vi "VIAn_EasyAnalyze.vi"(8 "error in (no error)":errorcluster, 11 "CommandLine":string[](array[string])) -> (0 "error out":errorcluster, 2 "test details":string, 3 "output to action":string)   [LabVIEW 2014]
uses:
  <userlib>/_OpenG.lib/string/string.llb/Trim Whitespace (String)__ogtk.vi
  _lvcicd/_lvcicd_support_2014.lvlib
  <vilib>/addons/analyzer/NI_VIAnalyzerTKVIs.lvlib
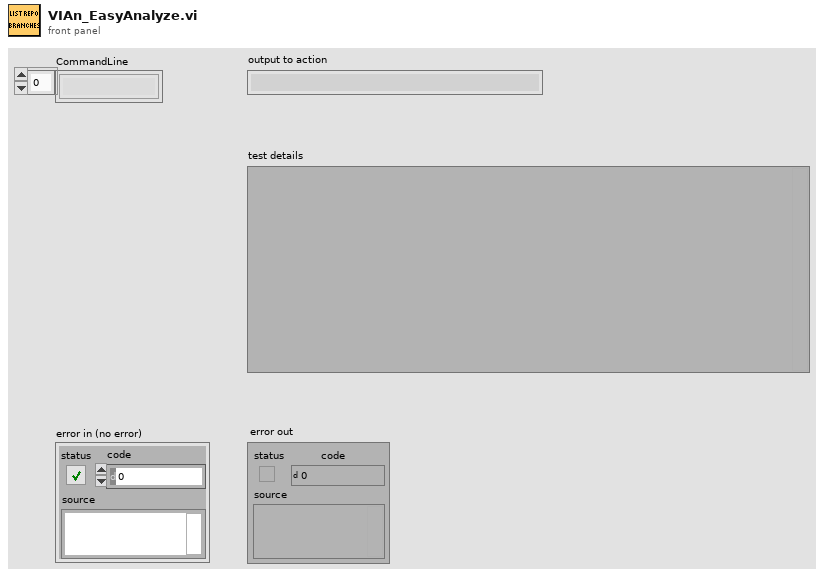
[diagram p1: front panel]
types:
  T1 = typedef "VIAnCtl Results.ctl" = cluster{"Test Name":string, "Results Data":T2[], "Status":T3, "Exceed Max Fails?":bool}
  T2 = typedef "VIAnCtl ResultsData (index).ctl" = cluster{"Result Message":string, "Ref Index":i32}
  T3 = typedef "VIAnCtl ResultStatus.ctl" = enum16{"Pass", "Fail", "Skipped", "VI not loadable", "Test not loadable", "Test not runnable", "Test error out"}
  T4 = typedef "VIAnRes Parsed Results Data (by VI).ctl" = cluster{"VI Path":path, "Pass":cluster{"row":i32, "column":i32}[], "Fail":cluster{"row":i32, "column":i32}[], "Skipped":cluster{"row":i32, "column":i32}[], "VI not loadable":cluster{"row":i32, "column":i32}[], "Test not loadable":cluster{"row":i32, "column":i32}[], "Test not runnable":cluster{"row":i32, "column":i32}[], "Test error out":cluster{"row":i32, "column":i32}[]}
  T5 = typedef "VIAnRes Parsed Results Data (by Test).ctl" = cluster{"Test Name":string, "Pass":cluster{"VI Path":path, "index":cluster{"row":i32, "column":i32}}[], "Fail":cluster{"VI Path":path, "index":cluster{"row":i32, "column":i32}}[], "Skipped":cluster{"VI Path":path, "index":cluster{"row":i32, "column":i32}}[]}
  T6 = typedef "VIAnCtl Test Config Data.ctl" = cluster{"Test Name":string, "Config Ref":refnum<vi>, "Ref Valid?":bool, "Test Ranking":T7, "Max Failures":u32, "Test Path":path, "Control Values":T8[], "Selected?":bool}
  T7 = typedef "VIAnCtl TestRanking.ctl" = u16
  T8 = typedef "VIAnCtl Config Control Value.ctl" = cluster{"Control Name":string, "Control Value":variant}
  T9 = cluster{"Raw Results":T1[][], "Parsed Results Data (by VI)":T4[], "Parsed Results Data (by Test)":T5[], "Summary Statistics":cluster{"Passed Tests":i32, "Failed Tests":i32, "Skipped Tests":i32, "VIs not loadable":i32, "Tests not loadable":i32, "Tests not runnable":i32, "Test error out":i32, "Start Time":u32, "Total Time (s)":dbl}, "Test Config Data":T6[]}
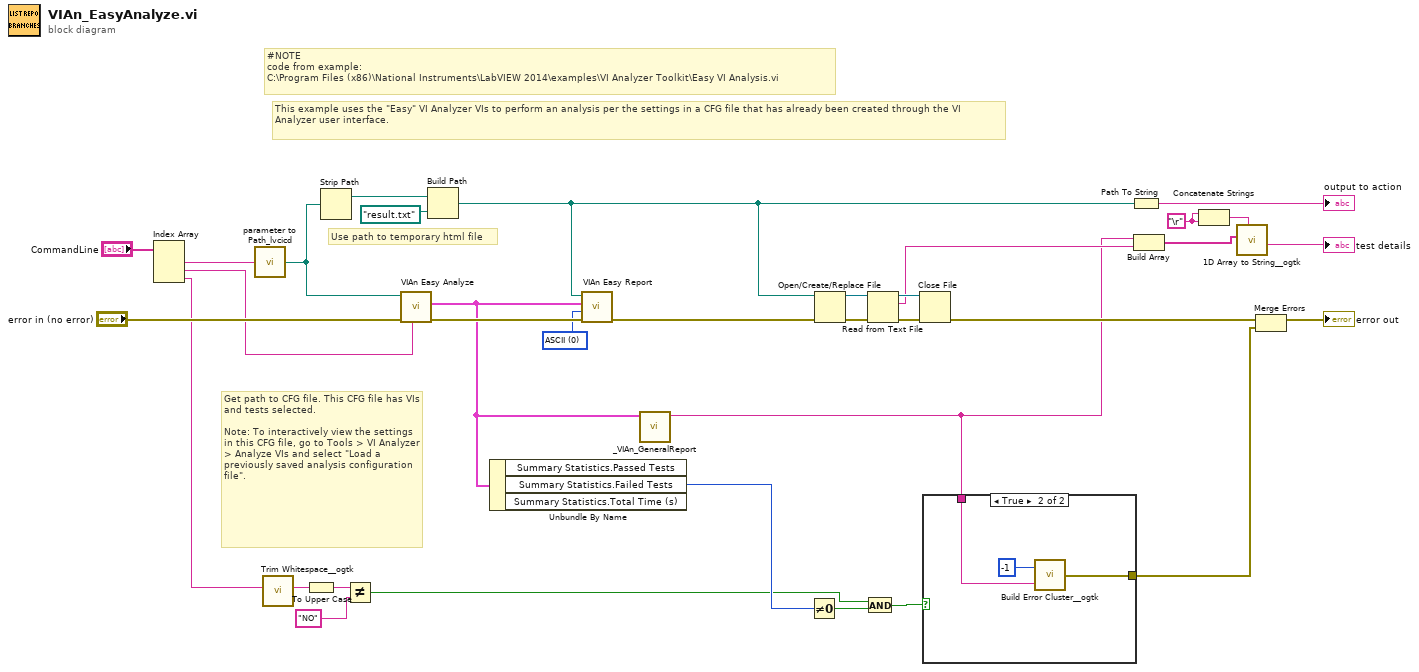
[diagram p0: block diagram]
diagram:
  w14 = "\r"
  w30 = u16 0 items=["ASCII", "HTML", "RSL File"] ("Report Save Type (ASCII)")
  # "#NOTE\ncode from example: \nC:\\Program Files (x86)\\National Instruments\\LabVIEW 2014\\examples\\VI Analyzer Toolkit\\Easy VI Analysis.vi"
  # "Use path to temporary html file"
  # "This example uses the \"Easy\" VI Analyzer VIs to perform an analysis per the settings in a CFG file that has already been created through the VI Analyzer user interface."
  # "Get path to CFG file. This CFG file has VIs and tests selected.\n \nNote: To interactively view the settings in this CFG file, go to Tools > VI Analyzer > Analyze VIs and select \"Load a previously saved analysis configuration file\"."
  n1 = Index Array(array="CommandLine") -> (element #1=w33:string, element #2=w20:string, element #3=w7:string)  [unwired: 3 in]
  n2 = call "parameter to Path_lvcicd.vi"("String"=w33) -> ("Path"=w19:path)
  n3 = call-poly <userlib>:"Trim Whitespace__ogtk.vi"("String in"=w7) -> ("String out"=w8:string)  [unwired: 6 in]
  n4 = To Upper Case(1:w8) -> (0:w9:string)
  n5 = Strip Path(path=w19) -> (stripped path=w18:path)  [unwired: 1 out]
  n6 = Not Equal?(x=w9, y="NO") -> (x != y?=w3:bool)
  n7 = call <vilib>:"VIAn Easy Analyze.vi"("Configuration File Password"=w20, "error in (no error)"="error in (no error)", "Analysis Target"=w19) -> ("error out"=w31:errorcluster, "Analysis Results"=w11:T9)  [unwired: 7 out]
  n8 = Build Path(base path=w18, name or relative path=path "result.txt" ("path")) -> (appended path=w17:path)
  n9 = Unbundle By Name(w11) -> ("Summary Statistics.Failed Tests"=w4:i32)  [unwired: 2 out]
  n10 = call <vilib>:"VIAn Easy Report.vi"("error in (no error)"=w31, "Report Save Type (ASCII)"=w30, "Analysis Results"=w11, "Report Save Path"=w17) -> ("error out"=w27:errorcluster)  [unwired: 3 in, 4 out]
  n11 = call "_VIAn_GeneralReport.vi"("Analysis Results"=w11) -> ("String"=w2:string)  [unwired: 7 in, 3 out]
  n12 = Not Equal To 0?(x=w4) -> (x != 0?=w6:bool)
  n13 = Open/Create/Replace File(file path (use dialog)=w17, error in=w27) -> (refnum out=w23:refnum<file>, error out=w25:errorcluster)  [unwired: 4 in, 1 out]
  n14 = And(x=w3, y=w6) -> (x .and. y?=w5:bool)
  n15 = Read from Text File(file (use dialog)=w23, error in=w25) -> (refnum out=w22:refnum<file>, text=w21:string, error out=w24:errorcluster)  [unwired: 2 in, 1 out]
  n16 = Close File(refnum=w22, error in=w24) -> (error out=w26:errorcluster)  [unwired: 1 out]
  n17 = case shown="True" w5 {
    tunnel: [_ w36] -> w1
    tunnel: w2 -> [_ w35]
    frame False {
    }
    frame True {
      n18 = call <userlib>:"Build Error Cluster__ogtk.vi"("String to Prepend to source (\"\")"=w35, "code"=-1) -> ("error out"=w36:errorcluster)
    }
  }
  n19 = Path To String(path=w17) -> (string=→"output to action":string)
  n20 = Build Array(w2, w21) -> (w13:string[])
  n21 = Concatenate Strings(w14, w14) -> (w15:string)
  n22 = call <userlib>:"1D Array to String__ogtk.vi"("delimiter (Tab)"=w15, "Array of Strings"=w13) -> ("delimited string"=→"test details":string)  [unwired: 9 in]
  n23 = Merge Errors(w26, w1) -> (→"error out":errorcluster)
